vi "Labspec LoadConfig.vi"(8 "error in":errorcluster, 9 "Path":path, 10 "ShowDialog":u16(ring) items=["Don't show the setup dialog", "Show the setup, load the configuration", "Show the setup, don't load the configuration"], 11 "Automation Refnum In":refnum<k7>) -> (0 "error out":errorcluster, 3 "Automation Refnum Out":refnum<k7>)   [LabVIEW 2014]
panel:
  # "LICENSED MATERIALS – PROPERTY OF IBM\nCopyright IBM Corp. 2016,\nALL RIGHTS RESERVED"
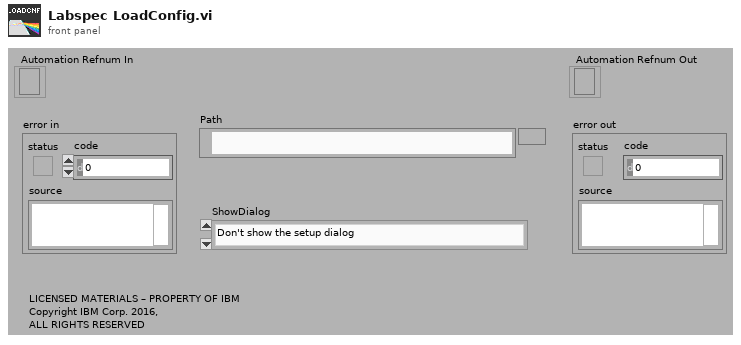
[diagram p1: front panel]
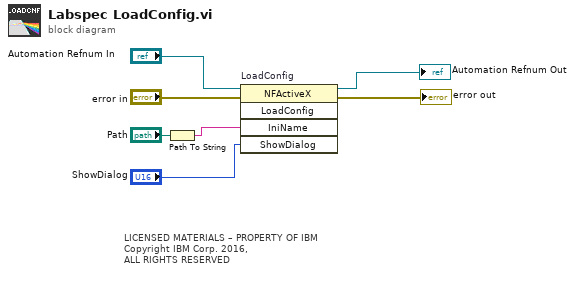
[diagram p0: block diagram]
diagram:
  # "LICENSED MATERIALS – PROPERTY OF IBM\nCopyright IBM Corp. 2016,\nALL RIGHTS RESERVED"
  n1 = Path To String(path="Path") -> (string=w2:string)
  n2 = invoke on="LoadConfig" class="NFActiveX" method="LoadConfig"(reference="Automation Refnum In", error in="error in", "IniName"=w2, "ShowDialog"="ShowDialog") -> (reference out=→"Automation Refnum Out":refnum<k7>, error out=→"error out":errorcluster)  [unwired: 1 in, 3 out]
